vi "Init TCP (Session).vi"(7 "Error Checking (Full)":T1=enum."Full", 8 "error in (no error)":errorcluster, 11 "VISA resource name":refnum<visa-resource-name>) -> (0 "error out":errorcluster, 3 "Session":refnum<class "Session.lvclass">)   [LabVIEW 2020, in "CTI.lvlib" / "VisaComms.lvclass"]
uses:
  VisaComms.lvclass
  Session/Session.lvclass
  Error Reporting.ctl
  C:/dev/cti/cti-drivers-lv-visa/CTI/DeviceComms/DeviceComms.lvclass
  <vilib>/Instr/_visa.llb/VISA Open Access Mode.ctl
  VisaComms.lvclass/VisaComms.ctl
  CTI.lvlib
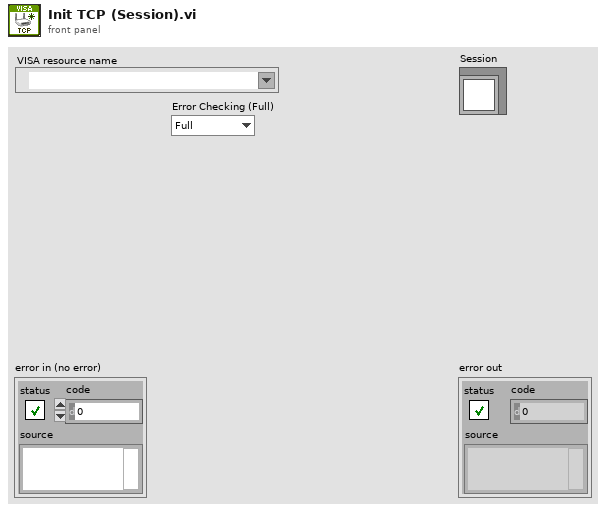
[diagram p1: front panel]
types:
  T1 = typedef "CTI.lvlib/Error Reporting.ctl" = enum16{"Minimal", "Moderate", "Full"}
  T2 = typedef "VISA Open Access Mode.ctl" = u32
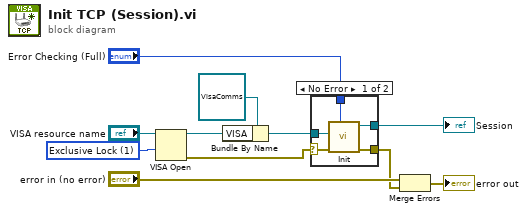
[diagram p0: block diagram]
diagram:
  w7 = T2 1 items=["VISA Defaults"=0, "Exclusive Lock"=1, "Load Configured Settings"=4] ("Access Mode")
  n1 = VISA Open(access mode=w7, VISA resource name="VISA resource name") -> (VISA resource name=w8:refnum<visa-resource-name>, error out=w5:errorcluster)  [unwired: 3 in]
  n2 = Bundle By Name(cluster=refnum<class "VisaComms.lvclass"> refnum ("CTI.lvlib:VisaComms.lvclass"), "VISA"=w8) -> (w6:refnum<class "VisaComms.lvclass">)
  n3 = case shown="No Error" w5 {
    selector: w5 -> [w13 w17]
    tunnel: [w16 _] -> w2
    tunnel: [w15 w17] -> w3
    tunnel: w6 -> [w14 _]
    tunnel: "Error Checking (Full)" -> [w12 _]
    frame No Error {
      n4 = call "Init.vi"("Error Checking (Full)"=w12, "error in (no error)"=w13, "DeviceComms"=w14) -> ("error out"=w15:errorcluster, "Session out"=w16:refnum<class "Session.lvclass">)  [unwired: 6 in, 1 out]
    }
    frame Error {
    }
  }
  "Session" <- w2
  n5 = Merge Errors("error in (no error)", w3) -> (→"error out":errorcluster)
